vi "Main.vi"(8 "error in (no error)":errorcluster, 11 "TomoBase in":refnum<class "Tomo.lvclass">) -> (0 "error out":errorcluster, 3 "component":refnum<class "Tomo.lvclass">)   [LabVIEW 2012, in "Tomo.lvclass"]
doc: "Main VI of the component."
uses:
  Tomo.lvclass
  <vilib>/Distrio/Murmex/Murmex/command_enum.ctl
  Tomo.lvclass/Tomo.ctl
  <vilib>/Distrio/Murmex/InitialiseMessage/InitialiseMessage.lvclass
  <vilib>/Distrio/Murmex/TerminateMessage/TerminateMessage.lvclass
  <vilib>/Distrio/Murmex/ConfigureMessage/ConfigureMessage.lvclass
  <vilib>/Distrio/Murmex/Murmex/update_cluster.ctl
  <vilib>/Distrio/Murmex/StopMessage/StopMessage.lvclass
  <vilib>/Distrio/Murmex/GenericMessage/GenericMessage.lvclass
  <vilib>/Distrio/Murmex/Murmex/Set configure at initialise.vi
  <vilib>/Distrio/Murmex/Murmex/Set log reference.vi
  <vilib>/Distrio/Murmex/Murmex/Set VI reference.vi
  <vilib>/Distrio/Murmex/Murmex/Set write log to disk.vi
  <vilib>/Distrio/Murmex/Message/Add or replace parameter.vi
  <vilib>/Distrio/Murmex/Murmex/Murmex.lvclass
  <vilib>/Distrio/Murmex/Message/Message.lvclass
panel:
  in  "Tab Control":T1(tab)
  out "TB":dbl format="%#_2g"
  out "Tomography progress":dbl(slide) scale=0.0..1.0
  in  "experiment name":string
  in  "Volume map":T2(ring)
  in  "Z step size":dbl[unit]=1e-06
  in  "X step size":dbl[unit]=0.0005
  in  "Y step size":dbl[unit]=0.0005
  in  "# of views":dbl=1.0
  in  "starting angle":dbl[unit]
  in  "button::start":bool
  out "Estimated remaining time":dbl format="- %<%H:%M:%S>t"
  in  "X min":dbl[unit]
  in  "X max":dbl[unit]
  in  "Y min":dbl[unit]
  in  "Y max":dbl[unit]
  in  "Z min":dbl[unit]
  in  "Z max":dbl[unit]
  in  "Pre tomo volume file":path
  in  "Pre tomo binary images path":path
  in  "button::pretomo calc":bool
  in  "Custom volume path":path
  in  "Experimenter email address":string
  in  "Experimenter name":string
  in  "generic command":string
  in  "button::send command":bool
  out "log":string
  in  "ID":string="tomo"
  in  "command":T3
  in  "recipient":string
  in  "button::configure":bool
  in  "button::quit":bool
  in  "terminate?":bool
  # "Tomo\n\nImplemented by:\nLudovico Silvestri\nUniversity of Florence, Italy"
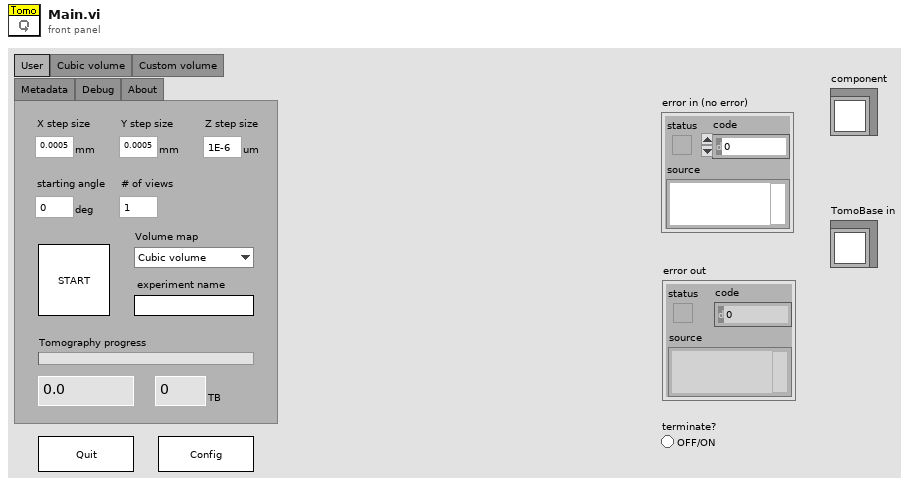
[diagram p1: front panel]
types:
  T1 = enum32{"User", "Cubic volume", "Custom volume", "Metadata", "Debug", "About"}
  T2 = enum16{"Cubic volume", "Custom volume", "Self-generate volume"}
  T3 = typedef "Murmex.lvlib/Murmex.lvclass/command_enum.ctl" = enum16{"null", "initialise", "reset", "terminate", "acknowledge", "update", "inspect", "inform", "proceed", "start", "stop", "fetch", "configure", "generic"}
  T4 = typedef "Murmex.lvlib/Murmex.lvclass/update_cluster.ctl" = cluster{"target ID":string, "key chains":string[], "values":variant[]}
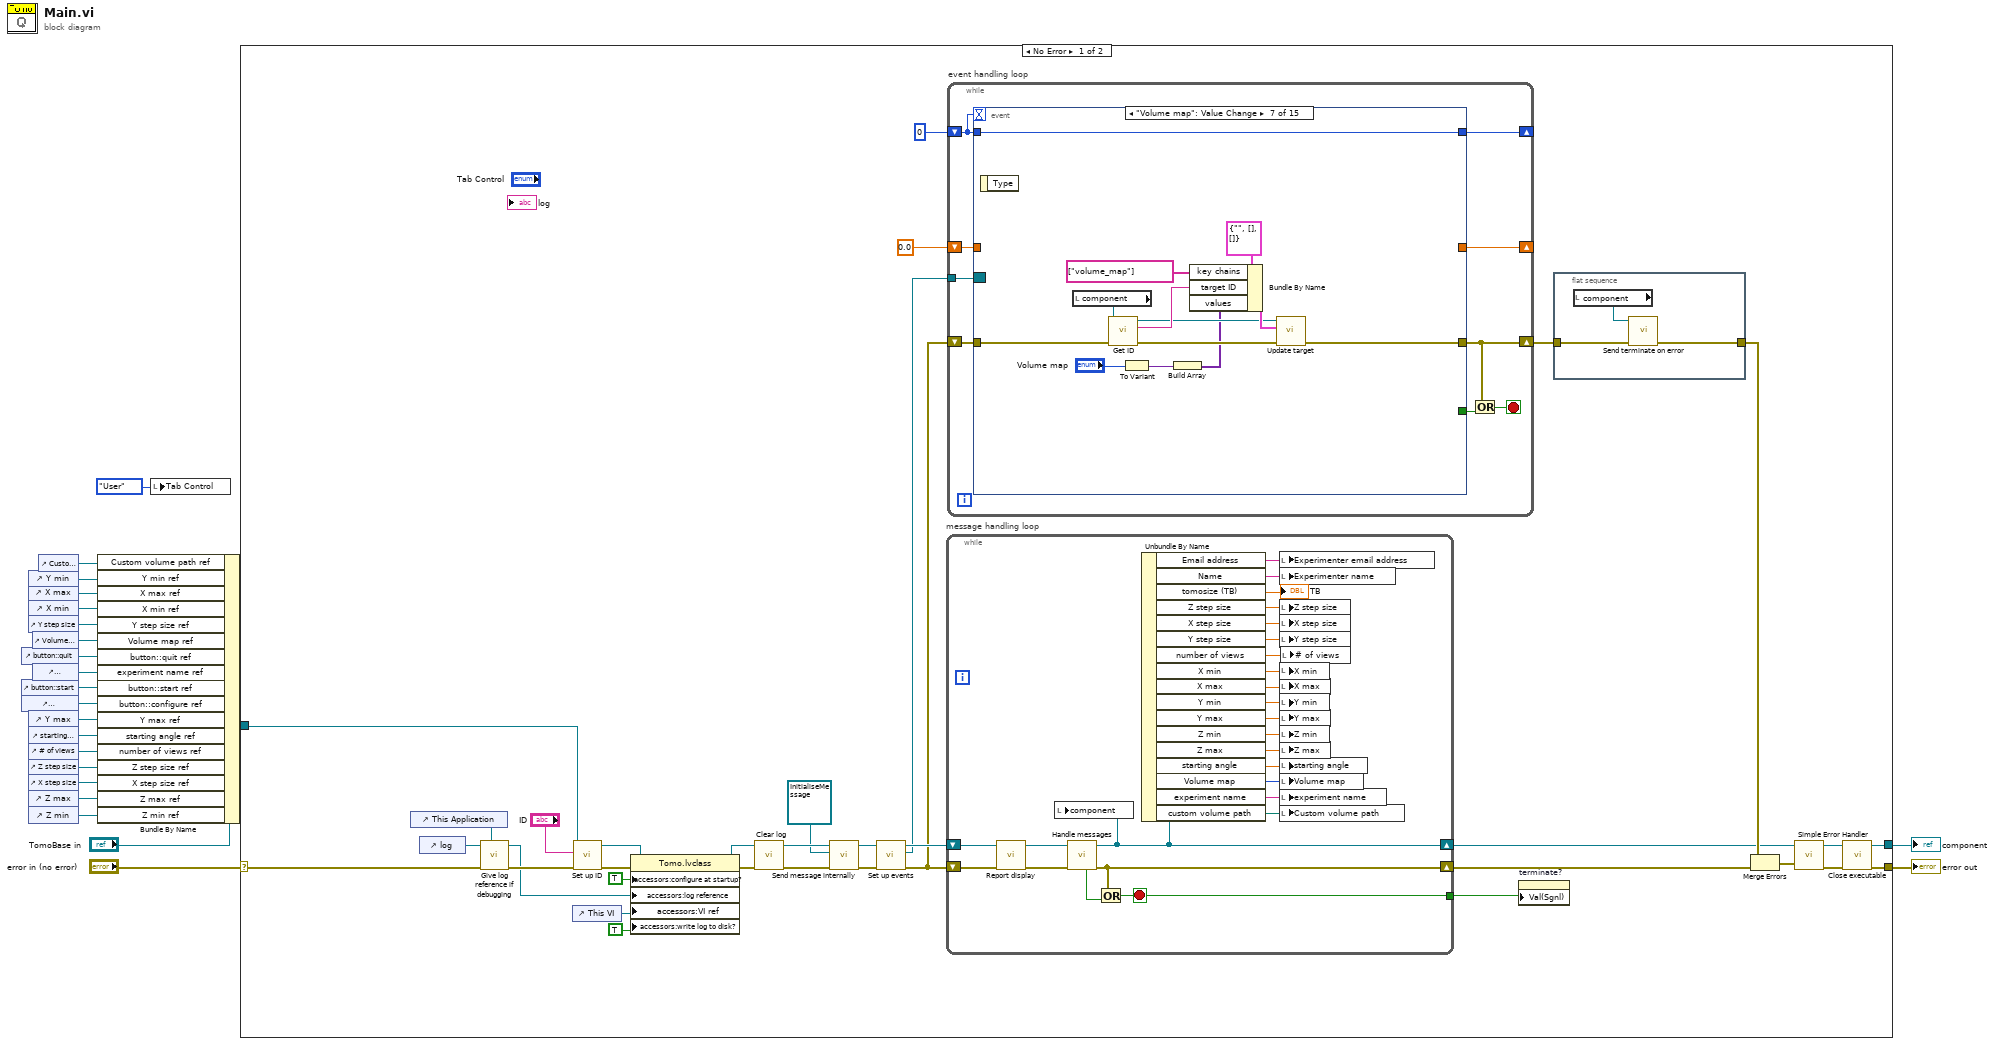
[diagram p0: block diagram]
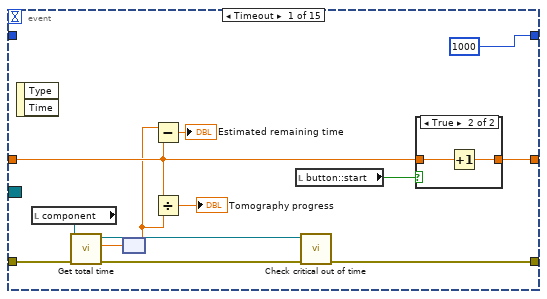
[diagram p2: hidden frame]
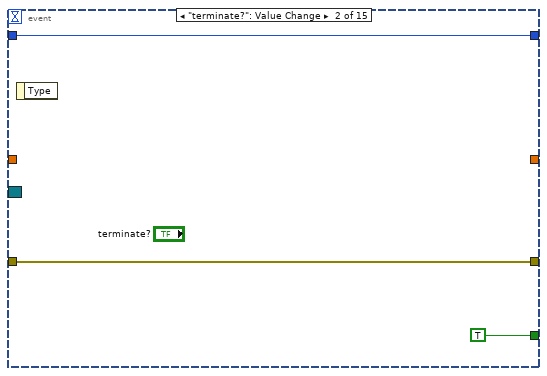
[diagram p4: hidden frame]
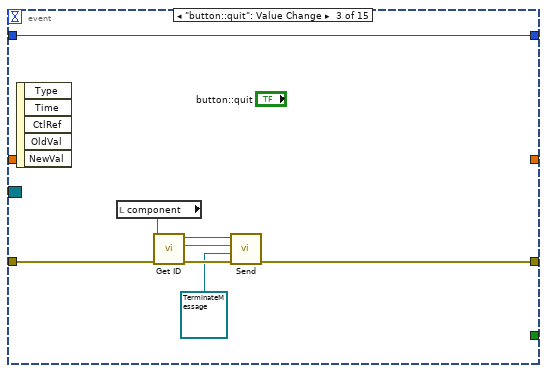
[diagram p5: hidden frame]
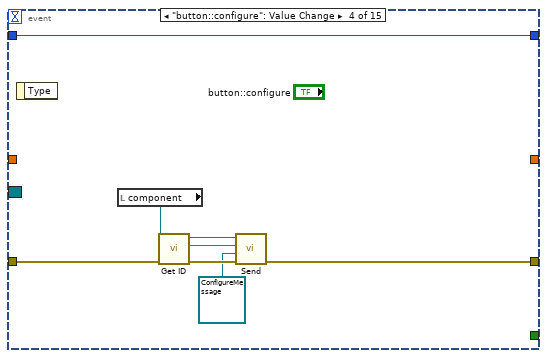
[diagram p6: hidden frame]
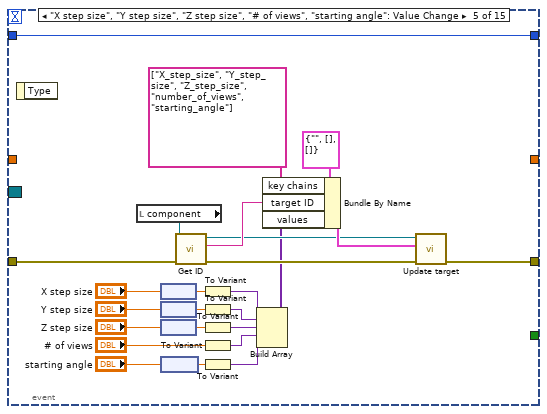
[diagram p7: hidden frame]
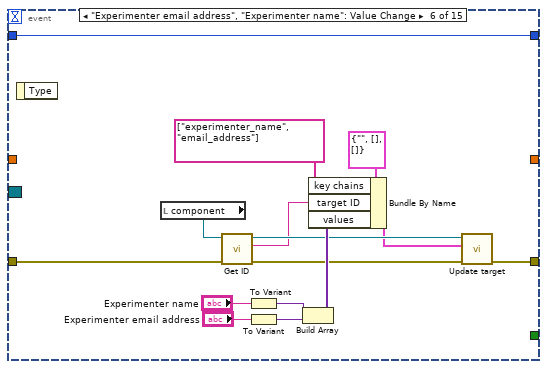
[diagram p8: hidden frame]
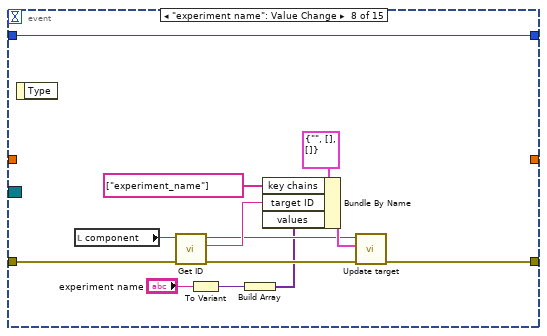
[diagram p9: hidden frame]
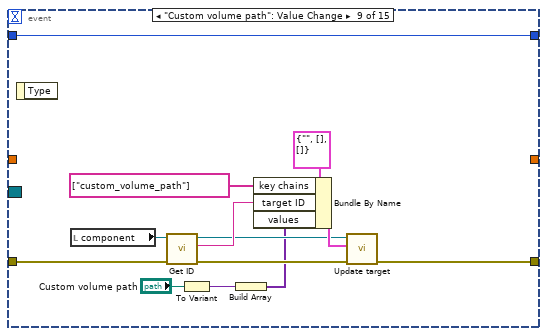
[diagram p10: hidden frame]
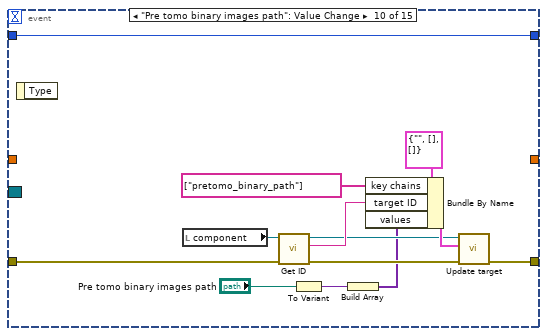
[diagram p11: hidden frame]
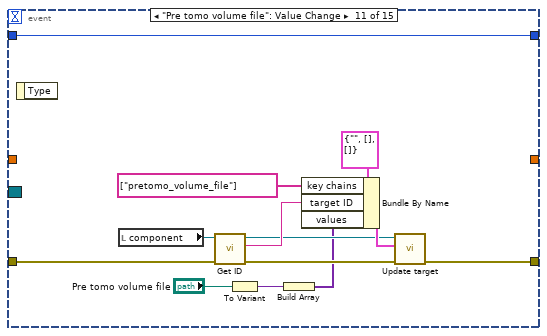
[diagram p12: hidden frame]
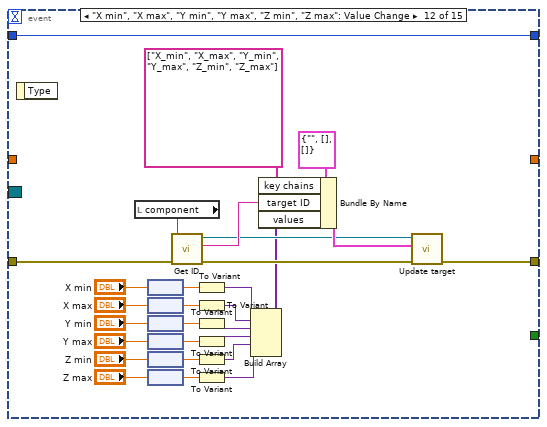
[diagram p13: hidden frame]
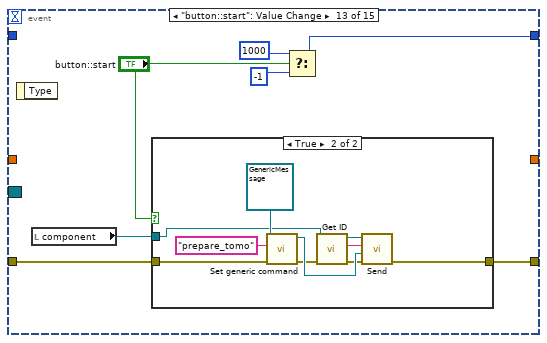
[diagram p14: hidden frame]
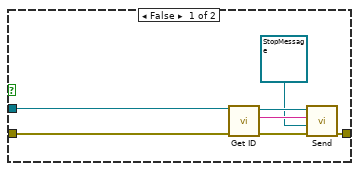
[diagram p15: hidden frame]
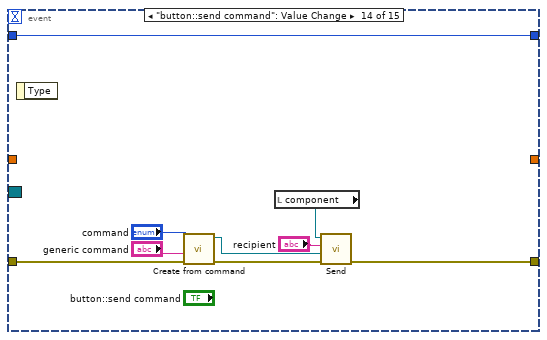
[diagram p16: hidden frame]
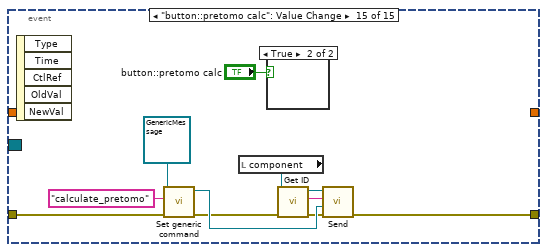
[diagram p17: hidden frame]
diagram:
  n1 = control-ref of="button::quit"() -> (w12:refnum<vi>)
  n2 = control-ref of="button::start"() -> (w10:refnum<vi>)
  n3 = control-ref of="button::configure"() -> (w9:refnum<vi>)
  n4 = control-ref of="Y min"() -> (w17:refnum<vi>)
  n5 = control-ref of="X max"() -> (w16:refnum<vi>)
  n6 = control-ref of="X min"() -> (w15:refnum<vi>)
  n7 = control-ref of="Y step size"() -> (w14:refnum<vi>)
  n8 = control-ref of="Y max"() -> (w8:refnum<vi>)
  n9 = control-ref of="starting angle"() -> (w7:refnum<vi>)
  n10 = control-ref of="# of views"() -> (w6:refnum<vi>)
  n11 = control-ref of="Z step size"() -> (w5:refnum<vi>)
  n12 = control-ref of="X step size"() -> (w4:refnum<vi>)
  n13 = control-ref of="Z max"() -> (w3:refnum<vi>)
  n14 = control-ref of="Z min"() -> (w2:refnum<vi>)
  n15 = control-ref of="Volume map"() -> (w13:refnum<vi>)
  n16 = control-ref of="experiment name"() -> (w11:refnum<vi>)
  n17 = control-ref of="Custom volume path"() -> (w18:refnum<vi>)
  n18 = Bundle By Name(cluster="TomoBase in", "Custom volume path ref"=w18, "Y min ref"=w17, "X max ref"=w16, "X min ref"=w15, "Y step size ref"=w14, "Volume map ref"=w13, "button::quit ref"=w12, "experiment name ref"=w11, "button::start ref"=w10, "button::configure ref"=w9, "Y max ref"=w8, "starting angle ref"=w7, "number of views ref"=w6, "Z step size ref"=w5, "X step size ref"=w4, "Z max ref"=w3, "Z min ref"=w2) -> (w19:refnum<class "Tomo.lvclass">)
  n19 = local write "Tab Control"(T1."User" ("Tab Control")) -> ()
  n20 = case shown="No Error" "error in (no error)" {
    selector: "error in (no error)" -> [w28 w307]
    tunnel: w19 -> [w53 w306]
    tunnel: [w33 w307] -> w22
    tunnel: [w31 w306] -> w21
    frame No Error {
      n21 = control-ref of="This Application"() -> (w25:refnum<vi>)
      n22 = control-ref of="log"() -> (w27:refnum<vi>)
      n23 = call "Give log reference if debugging.vi"("application ref"=w25, "error in (no error)"=w28, "log reference in"=w27) -> ("error out"=w29:errorcluster, "log reference out"=w26:refnum<vi>)  [unwired: 6 in, 1 out]
      n24 = control-ref of="This VI"() -> (w55:refnum<vi>)
      n25 = call <vilib>:"Set up ID.vi"("error in (no error)"=w29, "component ID"="ID", "MurmexBase in"=w53) -> ("error out"=w54:errorcluster, "MurmexBase out"=w51:refnum<class "Tomo.lvclass">)  [unwired: 6 in, 1 out]
      n26 = property class="Tomo.lvclass"(reference=w51, error in=w54, "accessors:configure at startup?"=TRUE ("configure at startup?"), "accessors:log reference"=w26, "accessors:VI ref"=w55, "accessors:write log to disk?"=TRUE ("write log to disk?")) -> (reference out=w49:refnum<class "Tomo.lvclass">, error out=w50:errorcluster)
      n27 = call <vilib>:"Clear log.vi"("error in (no error)"=w50, "MurmexBase in"=w49) -> ("error out"=w48:errorcluster, "MurmexBase out"=w47:refnum<class "Tomo.lvclass">)  [unwired: 8 in]
      n28 = call <vilib>:"Send message internally.vi"("error in (no error)"=w48, "Message"=refnum<class "InitialiseMessage.lvclass"> refnum ("Message in"), "Murmex in"=w47) -> ("error out"=w45:errorcluster, "Murmex out"=w44:refnum<class "Tomo.lvclass">)  [unwired: 7 in]
      n29 = call <vilib>:"Set up events.vi"("error in (no error)"=w45, "MurmexBase in"=w44) -> ("error out"=w42:errorcluster, "Event Registration Refnum"=w41:refnum<event-registration>, "MurmexBase out"=w43:refnum<class "Tomo.lvclass">)  [unwired: 7 in]
      n30 = while "message handling loop" {
        shift-right: [w286] -> w38
        shift-left: w42 -> [w284]
        shift-right: [w285] -> w32
        shift-left: w43 -> [w282]
        tunnel: [w304] -> w34
        stop <- w304 stop-if-true
        n31 = call-dynamic "Report display.vi"("error in (no error)"=w284, "Tomo in"=w282) -> ("error out"=w283:errorcluster, "Tomo out"=w281:refnum<class "Tomo.lvclass">)  [unwired: 8 in]
        n32 = call <vilib>:"Handle messages.vi"("error in (no error)"=w283, "Murmex in"=w281) -> ("error out"=w286:errorcluster, "Murmex out"=w285:refnum<class "Tomo.lvclass">, "terminated?"=w305:bool)  [unwired: 7 in]
        n33 = local write "component"(w285) -> ()
        n34 = Or(x=w286, y=w305) -> (x .or. y?=w304:bool)
        n35 = Unbundle By Name(w285) -> ("Email address"=w287:string, "Name"=w288:string, "tomosize (TB)"=→"TB":dbl, "Z step size"=w295:dbl[unit], "X step size"=w297:dbl[unit], "Y step size"=w296:dbl[unit], "number of views"=w294:dbl, "X min"=w303:dbl[unit], "X max"=w302:dbl[unit], "Y min"=w301:dbl[unit], "Y max"=w300:dbl[unit], "Z min"=w299:dbl[unit], "Z max"=w298:dbl[unit], "starting angle"=w293:dbl[unit], "Volume map"=w292:T2, "experiment name"=w291:string, "custom volume path"=w290:path)
        n36 = local write "Experimenter email address"(w287) -> ()
        n37 = local write "Experimenter name"(w288) -> ()
        n38 = local write "Z step size"(w295) -> ()
        n39 = local write "X step size"(w297) -> ()
        n40 = local write "Y step size"(w296) -> ()
        n41 = local write "X min"(w303) -> ()
        n42 = local write "X max"(w302) -> ()
        n43 = local write "Y min"(w301) -> ()
        n44 = local write "Y max"(w300) -> ()
        n45 = local write "Z min"(w299) -> ()
        n46 = local write "Z max"(w298) -> ()
        n47 = local write "starting angle"(w293) -> ()
        n48 = local write "Volume map"(w292) -> ()
        n49 = local write "experiment name"(w291) -> ()
        n50 = local write "Custom volume path"(w290) -> ()
        n51 = local write "# of views"(w294) -> ()
      }
      n52 = while "event handling loop" {
        shift-right: [w63] -> w39
        shift-left: w42 -> [w68]
        tunnel: w41 -> [w67]
        shift-right: [w65] -> _
        shift-left: 0 -> [w66]
        shift-right: [w60] -> _
        shift-left: 0.0 -> [w61]
        stop <- w62 stop-if-true
        n53 = event shown="[6] \"Volume map\": Value Change" {
          selector: w67 -> [_ _ _ _ _ _ _ _ _ _ _ _ _ _ _]
          dyn-events: _ -> [_ _ _ _ _ _ _ _ _ _ _ _ _ _ _]
          timeout: w66 -> [_ _ _ _ _ _ _ _ _ _ _ _ _ _ _]
          tunnel: [w70 w85 w92 w98 w126 w134 w150 w158 w174 w187 w200 w231 w243 w262 w271] -> w63
          tunnel: w68 -> [w81 w85 w94 w99 w124 w133 w152 w161 w173 w186 w199 w229 w242 w268 w272]
          tunnel: w66 -> [_ w84 w87 w95 w107 w128 w149 w157 w169 w183 w196 w215 _ w261 _]
          tunnel: [1000 w84 w87 w95 w107 w128 w149 w157 w169 w183 w196 w215 w237 w261 _] -> w65
          tunnel: [_ TRUE _ _ _ _ _ _ _ _ _ _ _ _ _] -> w64
          tunnel: w61 -> [w79 _ _ _ _ _ _ _ _ _ _ _ _ _ _]
          tunnel: [w78 _ _ _ _ _ _ _ _ _ _ _ _ _ _] -> w60
          event Timeout {
            n54 = event-data() -> ()  [unwired: 1 in, 2 out]
            n55 = local read "component"() -> (w77:refnum<class "Tomo.lvclass">)
            n56 = call-dynamic "Get total time.vi"("error in (no error)"=w81, "Tomo in"=w77) -> ("error out"=w80:errorcluster, "Total time"=w76:dbl[unit], "Tomo out"=w69:refnum<class "Tomo.lvclass">)  [unwired: 7 in]
            n57 = node(w76) -> (w74:dbl)
            n58 = Subtract(x=w74, y=w79) -> (x-y=→"Estimated remaining time":dbl)
            n59 = Divide(x=w79, y=w74) -> (x/y=→"Tomography progress":dbl)
            n60 = local read "button::start"() -> (w71:bool)
            n61 = call-dynamic "Check critical out of time.vi"("error in (no error)"=w80, "Tomo in"=w69) -> ("error out"=w70:errorcluster)  [unwired: 8 in, 1 out]
            n62 = case shown="True" w71 {
              tunnel: w79 -> [_ w83]
              tunnel: [_ w82] -> w78
              frame False {
              }
              frame True {
                n63 = Increment(x=w83) -> (x+1=w82:dbl)
              }
            }
          }
          event "terminate?": Value Change {
            n64 = event-data() -> ()  [unwired: 1 in, 1 out]
          }
          event "button::quit": Value Change {
            n65 = event-data() -> ()  [unwired: 1 in, 5 out]
            n66 = local read "component"() -> (w91:refnum<class "Tomo.lvclass">)
            n67 = call <vilib>:"Get ID.vi"("error in (no error)"=w94, "Murmex in"=w91) -> ("error out"=w93:errorcluster, "component id"=w89:string, "Murmex out"=w90:refnum<class "Tomo.lvclass">)  [unwired: 7 in]
            n68 = call <vilib>:"Send.vi"("error in (no error)"=w93, "Message"=refnum<class "TerminateMessage.lvclass"> refnum ("Distrio Murmex 1.1:TerminateMessage"), "recipient"=w89, "Murmex in"=w90) -> ("error out"=w92:errorcluster)  [unwired: 6 in, 1 out]
          }
          event "button::configure": Value Change {
            n69 = event-data() -> ()  [unwired: 1 in, 1 out]
            n70 = local read "component"() -> (w97:refnum<class "Tomo.lvclass">)
            n71 = call <vilib>:"Get ID.vi"("error in (no error)"=w99, "Murmex in"=w97) -> ("error out"=w102:errorcluster, "component id"=w100:string, "Murmex out"=w101:refnum<class "Tomo.lvclass">)  [unwired: 7 in]
            n72 = call <vilib>:"Send.vi"("error in (no error)"=w102, "Message"=refnum<class "ConfigureMessage.lvclass"> refnum ("Distrio Murmex 1.1:ConfigureMessage"), "recipient"=w100, "Murmex in"=w101) -> ("error out"=w98:errorcluster)  [unwired: 6 in, 1 out]
          }
          event "X step size", "Y step size", "Z step size", "# of views", "starting angle": Value Change {
            n73 = event-data() -> ()  [unwired: 1 in, 1 out]
            n74 = local read "component"() -> (w122:refnum<class "Tomo.lvclass">)
            n75 = node("X step size") -> (w106:dbl)
            n76 = node("Y step size") -> (w105:dbl)
            n77 = node("Z step size") -> (w104:dbl)
            n78 = node("starting angle") -> (w103:dbl)
            n79 = call <vilib>:"Get ID.vi"("error in (no error)"=w124, "Murmex in"=w122) -> ("error out"=w125:errorcluster, "component id"=w123:string, "Murmex out"=w120:refnum<class "Tomo.lvclass">)  [unwired: 7 in]
            n80 = To Variant(anything=w106) -> (Variant=w110:variant)
            n81 = To Variant(anything=w105) -> (Variant=w111:variant)
            n82 = To Variant(anything=w104) -> (Variant=w114:variant)
            n83 = To Variant(anything="# of views") -> (Variant=w113:variant)
            n84 = To Variant(anything=w103) -> (Variant=w112:variant)
            n85 = Build Array(w110, w111, w114, w113, w112) -> (w109:variant[])
            n86 = Bundle By Name(cluster=T4 {"target ID"="", "key chains"=[], "values"=[]} ("update cluster"), "key chains"=string[] ["X_step_size", "Y_step_size", "Z_step_size", "number_of_views", "starting_angle"], "target ID"=w123, "values"=w109) -> (w121:T4)
            n87 = call <vilib>:"Update target.vi"("error in (no error)"=w125, "update cluster"=w121, "MurmexBase in"=w120) -> ("error out"=w126:errorcluster)  [unwired: 7 in, 1 out]
          }
          event "Experimenter email address", "Experimenter name": Value Change {
            n88 = event-data() -> ()  [unwired: 1 in, 1 out]
            n89 = local read "component"() -> (w129:refnum<class "Tomo.lvclass">)
            n90 = call <vilib>:"Get ID.vi"("error in (no error)"=w133, "Murmex in"=w129) -> ("error out"=w136:errorcluster, "component id"=w137:string, "Murmex out"=w139:refnum<class "Tomo.lvclass">)  [unwired: 7 in]
            n91 = To Variant(anything="Experimenter name") -> (Variant=w141:variant)
            n92 = To Variant(anything="Experimenter email address") -> (Variant=w140:variant)
            n93 = Build Array(w141, w140) -> (w142:variant[])
            n94 = Bundle By Name(cluster=T4 {"target ID"="", "key chains"=[], "values"=[]} ("update cluster"), "key chains"=string[] ["experimenter_name", "email_address"], "target ID"=w137, "values"=w142) -> (w138:T4)
            n95 = call <vilib>:"Update target.vi"("error in (no error)"=w136, "update cluster"=w138, "MurmexBase in"=w139) -> ("error out"=w134:errorcluster)  [unwired: 7 in, 1 out]
          }
          event "Volume map": Value Change {
            n96 = event-data() -> ()  [unwired: 1 in, 1 out]
            n97 = local read "component"() -> (w143:refnum<class "Tomo.lvclass">)
            n98 = call <vilib>:"Get ID.vi"("error in (no error)"=w152, "Murmex in"=w143) -> ("error out"=w151:errorcluster, "component id"=w155:string, "Murmex out"=w153:refnum<class "Tomo.lvclass">)  [unwired: 7 in]
            n99 = To Variant(anything="Volume map") -> (Variant=w148:variant)
            n100 = Build Array(w148) -> (w147:variant[])
            n101 = Bundle By Name(cluster=T4 {"target ID"="", "key chains"=[], "values"=[]} ("update cluster"), "key chains"=string[] ["volume_map"], "target ID"=w155, "values"=w147) -> (w154:T4)
            n102 = call <vilib>:"Update target.vi"("error in (no error)"=w151, "update cluster"=w154, "MurmexBase in"=w153) -> ("error out"=w150:errorcluster)  [unwired: 7 in, 1 out]
          }
          event "experiment name": Value Change {
            n103 = event-data() -> ()  [unwired: 1 in, 1 out]
            n104 = local read "component"() -> (w156:refnum<class "Tomo.lvclass">)
            n105 = call <vilib>:"Get ID.vi"("error in (no error)"=w161, "Murmex in"=w156) -> ("error out"=w165:errorcluster, "component id"=w168:string, "Murmex out"=w166:refnum<class "Tomo.lvclass">)  [unwired: 7 in]
            n106 = To Variant(anything="experiment name") -> (Variant=w164:variant)
            n107 = Build Array(w164) -> (w163:variant[])
            n108 = Bundle By Name(cluster=T4 {"target ID"="", "key chains"=[], "values"=[]} ("update cluster"), "key chains"=string[] ["experiment_name"], "target ID"=w168, "values"=w163) -> (w167:T4)
            n109 = call <vilib>:"Update target.vi"("error in (no error)"=w165, "update cluster"=w167, "MurmexBase in"=w166) -> ("error out"=w158:errorcluster)  [unwired: 7 in, 1 out]
          }
          event "Custom volume path": Value Change {
            n110 = event-data() -> ()  [unwired: 1 in, 1 out]
            n111 = local read "component"() -> (w171:refnum<class "Tomo.lvclass">)
            n112 = call <vilib>:"Get ID.vi"("error in (no error)"=w173, "Murmex in"=w171) -> ("error out"=w178:errorcluster, "component id"=w181:string, "Murmex out"=w179:refnum<class "Tomo.lvclass">)  [unwired: 7 in]
            n113 = To Variant(anything="Custom volume path") -> (Variant=w177:variant)
            n114 = Build Array(w177) -> (w176:variant[])
            n115 = Bundle By Name(cluster=T4 {"target ID"="", "key chains"=[], "values"=[]} ("update cluster"), "key chains"=string[] ["custom_volume_path"], "target ID"=w181, "values"=w176) -> (w180:T4)
            n116 = call <vilib>:"Update target.vi"("error in (no error)"=w178, "update cluster"=w180, "MurmexBase in"=w179) -> ("error out"=w174:errorcluster)  [unwired: 7 in, 1 out]
          }
          event "Pre tomo binary images path": Value Change {
            n117 = event-data() -> ()  [unwired: 1 in, 1 out]
            n118 = local read "component"() -> (w185:refnum<class "Tomo.lvclass">)
            n119 = call <vilib>:"Get ID.vi"("error in (no error)"=w186, "Murmex in"=w185) -> ("error out"=w191:errorcluster, "component id"=w194:string, "Murmex out"=w192:refnum<class "Tomo.lvclass">)  [unwired: 7 in]
            n120 = To Variant(anything="Pre tomo binary images path") -> (Variant=w190:variant)
            n121 = Build Array(w190) -> (w189:variant[])
            n122 = Bundle By Name(cluster=T4 {"target ID"="", "key chains"=[], "values"=[]} ("update cluster"), "key chains"=string[] ["pretomo_binary_path"], "target ID"=w194, "values"=w189) -> (w193:T4)
            n123 = call <vilib>:"Update target.vi"("error in (no error)"=w191, "update cluster"=w193, "MurmexBase in"=w192) -> ("error out"=w187:errorcluster)  [unwired: 7 in, 1 out]
          }
          event "Pre tomo volume file": Value Change {
            n124 = event-data() -> ()  [unwired: 1 in, 1 out]
            n125 = local read "component"() -> (w198:refnum<class "Tomo.lvclass">)
            n126 = call <vilib>:"Get ID.vi"("error in (no error)"=w199, "Murmex in"=w198) -> ("error out"=w204:errorcluster, "component id"=w207:string, "Murmex out"=w205:refnum<class "Tomo.lvclass">)  [unwired: 7 in]
            n127 = To Variant(anything="Pre tomo volume file") -> (Variant=w203:variant)
            n128 = Build Array(w203) -> (w202:variant[])
            n129 = Bundle By Name(cluster=T4 {"target ID"="", "key chains"=[], "values"=[]} ("update cluster"), "key chains"=string[] ["pretomo_volume_file"], "target ID"=w207, "values"=w202) -> (w206:T4)
            n130 = call <vilib>:"Update target.vi"("error in (no error)"=w204, "update cluster"=w206, "MurmexBase in"=w205) -> ("error out"=w200:errorcluster)  [unwired: 7 in, 1 out]
          }
          event "X min", "X max", "Y min", "Y max", "Z min", "Z max": Value Change {
            n131 = event-data() -> ()  [unwired: 1 in, 1 out]
            n132 = local read "component"() -> (w228:refnum<class "Tomo.lvclass">)
            n133 = node("X min") -> (w214:dbl)
            n134 = node("X max") -> (w213:dbl)
            n135 = node("Y min") -> (w212:dbl)
            n136 = node("Y max") -> (w211:dbl)
            n137 = node("Z min") -> (w209:dbl)
            n138 = node("Z max") -> (w208:dbl)
            n139 = call <vilib>:"Get ID.vi"("error in (no error)"=w229, "Murmex in"=w228) -> ("error out"=w230:errorcluster, "component id"=w235:string, "Murmex out"=w233:refnum<class "Tomo.lvclass">)  [unwired: 7 in]
            n140 = To Variant(anything=w214) -> (Variant=w224:variant)
            n141 = To Variant(anything=w213) -> (Variant=w225:variant)
            n142 = To Variant(anything=w212) -> (Variant=w227:variant)
            n143 = To Variant(anything=w211) -> (Variant=w226:variant)
            n144 = To Variant(anything=w209) -> (Variant=w217:variant)
            n145 = To Variant(anything=w208) -> (Variant=w216:variant)
            n146 = Build Array(w224, w225, w227, w226, w217, w216) -> (w223:variant[])
            n147 = Bundle By Name(cluster=T4 {"target ID"="", "key chains"=[], "values"=[]} ("update cluster"), "key chains"=string[] ["X_min", "X_max", "Y_min", "Y_max", "Z_min", "Z_max"], "target ID"=w235, "values"=w223) -> (w234:T4)
            n148 = call <vilib>:"Update target.vi"("error in (no error)"=w230, "update cluster"=w234, "MurmexBase in"=w233) -> ("error out"=w231:errorcluster)  [unwired: 7 in, 1 out]
          }
          event "button::start": Value Change {
            n149 = event-data() -> ()  [unwired: 1 in, 1 out]
            n150 = local read "component"() -> (w241:refnum<class "Tomo.lvclass">)
            n151 = case shown="True" "button::start" {
              tunnel: [w248 w251] -> w243
              tunnel: w242 -> [w246 w253]
              tunnel: w241 -> [w244 w252]
              frame False {
                n152 = call <vilib>:"Get ID.vi"("error in (no error)"=w246, "Murmex in"=w244) -> ("error out"=w247:errorcluster, "component id"=w249:string, "Murmex out"=w250:refnum<class "Tomo.lvclass">)  [unwired: 7 in]
                n153 = call <vilib>:"Send.vi"("error in (no error)"=w247, "Message"=refnum<class "StopMessage.lvclass"> refnum ("Distrio Murmex 1.1:StopMessage"), "recipient"=w249, "Murmex in"=w250) -> ("error out"=w248:errorcluster)  [unwired: 6 in, 1 out]
              }
              frame True {
                n154 = call <vilib>:"Set generic command.vi"("error in (no error)"=w253, "generic command"="prepare_tomo", "GenericMessage in"=refnum<class "GenericMessage.lvclass"> refnum ("Message in")) -> ("error out"=w255:errorcluster, "GenericMessage out"=w259:refnum<class "GenericMessage.lvclass">)  [unwired: 7 in]
                n155 = call <vilib>:"Get ID.vi"("error in (no error)"=w255, "Murmex in"=w252) -> ("error out"=w256:errorcluster, "component id"=w258:string, "Murmex out"=w257:refnum<class "Tomo.lvclass">)  [unwired: 7 in]
                n156 = call <vilib>:"Send.vi"("error in (no error)"=w256, "Message"=w259, "recipient"=w258, "Murmex in"=w257) -> ("error out"=w251:errorcluster)  [unwired: 6 in, 1 out]
              }
            }
            n157 = Select(t=1000, s="button::start", f=-1) -> (s? t:f=w237:i32)
          }
          event "button::send command": Value Change {
            n158 = event-data() -> ()  [unwired: 1 in, 1 out]
            n159 = call <vilib>:"Create from command.vi"("error in (no error)"=w268, "generic command"="generic command", "command"="command") -> ("error out"=w263:errorcluster, "Message out"=w264:refnum<class "Message.lvclass">)  [unwired: 7 in]
            n160 = local read "component"() -> (w265:refnum<class "Tomo.lvclass">)
            n161 = call <vilib>:"Send.vi"("error in (no error)"=w263, "Message"=w264, "recipient"="recipient", "Murmex in"=w265) -> ("error out"=w262:errorcluster)  [unwired: 6 in, 1 out]
          }
          event "button::pretomo calc": Value Change {
            n162 = event-data() -> ()  [unwired: 1 in, 5 out]
            n163 = call <vilib>:"Set generic command.vi"("error in (no error)"=w272, "generic command"="calculate_pretomo", "GenericMessage in"=refnum<class "GenericMessage.lvclass"> refnum ("Message in")) -> ("error out"=w274:errorcluster, "GenericMessage out"=w278:refnum<class "GenericMessage.lvclass">)  [unwired: 7 in]
            n164 = local read "component"() -> (w270:refnum<class "Tomo.lvclass">)
            n165 = case shown="True" "button::pretomo calc" {
              frame False {
              }
              frame True {
              }
            }
            n166 = call <vilib>:"Get ID.vi"("error in (no error)"=w274, "Murmex in"=w270) -> ("error out"=w275:errorcluster, "component id"=w277:string, "Murmex out"=w276:refnum<class "Tomo.lvclass">)  [unwired: 7 in]
            n167 = call <vilib>:"Send.vi"("error in (no error)"=w275, "Message"=w278, "recipient"=w277, "Murmex in"=w276) -> ("error out"=w271:errorcluster)  [unwired: 6 in, 1 out]
          }
        }
        n168 = Or(x=w63, y=w64) -> (x .or. y?=w62:bool)
      }
      n169 = property on="terminate?" class="Bool (strict)"("Val(Sgnl)"=w34) -> ()  [unwired: 2 in, 2 out]
      n170 = flat-sequence {
        tunnel: w39 -> [w59]
        tunnel: [w57] -> w37
        frame #0 {
          n171 = local read "component"() -> (w58:refnum<class "Tomo.lvclass">)
          n172 = call <vilib>:"Send terminate on error.vi"("error in (no error)"=w59, "Murmex in"=w58) -> ("error out"=w57:errorcluster)  [unwired: 8 in, 1 out]
        }
      }
      n173 = Merge Errors(w37, w38) -> (w36:errorcluster)
      n174 = call <vilib>:"Simple Error Handler.vi"("error in (no error)"=w36) -> ("error out"=w35:errorcluster)  [unwired: 4 in, 4 out]
      n175 = call <vilib>:"Close executable.vi"("error in (no error)"=w35, "MurmexBase in"=w32) -> ("error out"=w33:errorcluster, "MurmexBase out"=w31:refnum<class "Tomo.lvclass">)  [unwired: 8 in]
    }
    frame Error {
    }
  }
  "error out" <- w22
  "component" <- w21
